vi "ArrayConcat.vi"() -> ()   [LabVIEW 2015]
panel:
  out "transposed array":dbl[][](array[numeric])=[[143423.0, 567.0, 124.0, 64.0, 0.0, 0.0, 123.0, 424.0, 234.0, 98.0, 124.0], [65467.0, 123.0, 346.0, 123.0, 0.0, 0.0, 453.0, 867.0, 75.0, 123.0, 881.0]]
  out "appended array 4":dbl[](array[numeric])=[124.0, 881.0, 124.0, 881.0]
  out "appended array 6":dbl[][](array[numeric])=[[143423.0, 65467.0], [567.0, 123.0], [124.0, 346.0], [64.0, 123.0], [0.0, 0.0], [0.0, 0.0], [123.0, 453.0], [424.0, 867.0], [234.0, 75.0], [98.0, 123.0], [124.0, 881.0]]
  in  "appended array 5":dbl[][](array[numeric])=[[143423.0, 65467.0], [567.0, 123.0], [124.0, 346.0], [64.0, 123.0], [0.0, 0.0], [0.0, 0.0], [123.0, 453.0], [424.0, 867.0], [234.0, 75.0], [98.0, 123.0]]
  in  "element 8":dbl=881.0
  in  "element 7":dbl=124.0
  out "appended array 3":dbl[](array[numeric])=[34655.0, 865.0, 875.0, 258954.0, 765.0, 6754.0]
  in  "element 6":dbl=258954.0
  in  "element 5":dbl=765.0
  out "appended array 2":dbl[](array[numeric])=[258954.0, 765.0, 6754.0]
  in  "element 4":dbl=6754.0
  in  "element 3":dbl=875.0
  out "appended array":dbl[](array[numeric])=[34655.0, 865.0, 875.0]
  in  "element 2":dbl=865.0
  in  "element":dbl=34655.0
  out "Ultimo Valor":dbl=2.1250089067969324
  out "Array":dbl[](array[numeric])=[4.595867222000216, 3.0188373432448112, 4.791093671089976, 4.326319107162405, 2.5524044072426473, 1.0179391315753272, 3.7719386668970465, 3.480425590873142, 4.830032474800305, 2.1250089067969324]
  out "Iteracion":i32=9
  out "Instantaneo":dbl=2.1250089067969324
  # "Union de Arreglos"
  # "Serrano Bermúdez Luis Esteban\nFecha de Entrega 17/02/2019"
  # "Descripcion: Esta aplicacion une varios elementos en arreglos o arreglos\nen un solo arrglo para crear matrices de elementos"
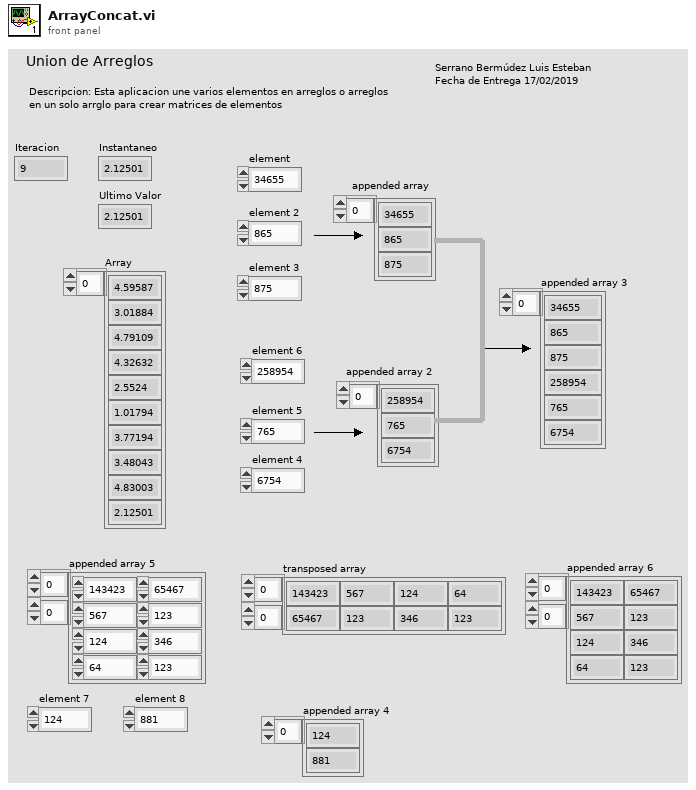
[diagram p1: front panel]
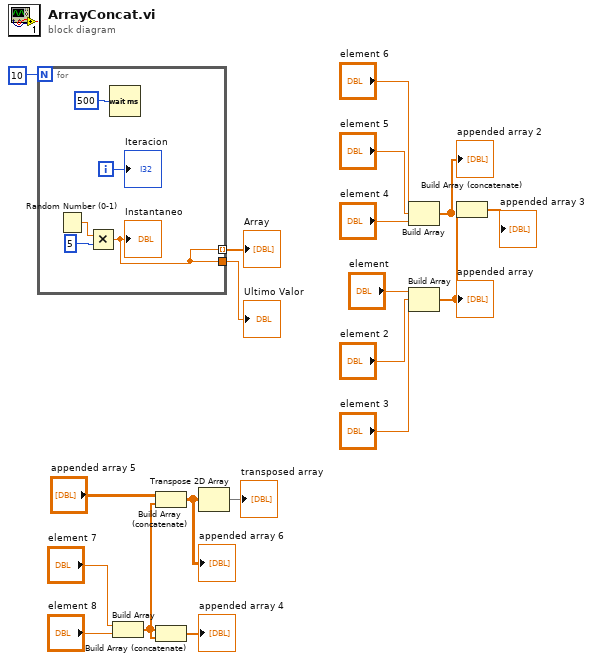
[diagram p0: block diagram]
diagram:
  n1 = for {
    N: 10 -> [_]
    tunnel: [w20] -> w18 mode=indexing
    tunnel: [w20] -> w17
    i -> [w21]
    n2 = Random Number (0-1)() -> (number: 0 to 1=w24:dbl)
    n3 = Multiply(x=w24, y=5) -> (x*y=w20:dbl)
    "Instantaneo" <- w20
    n4 = Wait (ms)(milliseconds to wait=u32 500) -> ()  [unwired: 1 out]
    "Iteracion" <- w21
  }
  "Array" <- w18
  "Ultimo Valor" <- w17
  n5 = Build Array("element 7", "element 8") -> (w5:dbl[])
  n6 = Build Array (concatenate)("appended array 5", w5) -> (w1:dbl[][])
  "appended array 6" <- w1
  n7 = Build Array (concatenate)(w5, w5) -> (→"appended array 4":dbl[])
  n8 = Transpose 2D Array(2D array=w1) -> (transposed array=→"transposed array":dbl[][])
  n9 = Build Array("element 6", "element 5", "element 4") -> (w9:dbl[])
  "appended array 2" <- w9
  n10 = Build Array("element", "element 2", "element 3") -> (w10:dbl[])
  "appended array" <- w10
  n11 = Build Array (concatenate)(w10, w9) -> (→"appended array 3":dbl[])
